vi "Initialize.vi"(8 "error in (no error)":errorcluster, 9 "Time":timestamp, 10 "Alias":string, 11 "NI DMM Calibration Data in":refnum<class "NI DMM Calibration Data.lvclass">) -> (0 "error out":errorcluster, 3 "NI DMM Calibration Data out":refnum<class "NI DMM Calibration Data.lvclass">)   [LabVIEW 2020, in "NI DMM Driver.lvlib" / "NI DMM Calibration Data.lvclass"]
doc: "Write Alias and Time and set all other values to NaN or FALSE."
uses:
  NI DMM Calibration Data.lvclass
  NI DMM Calibration Data.lvclass/NI DMM Calibration Data.ctl
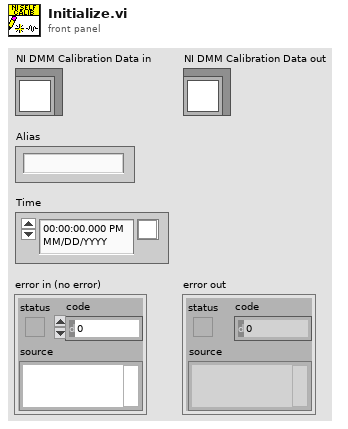
[diagram p1: front panel]
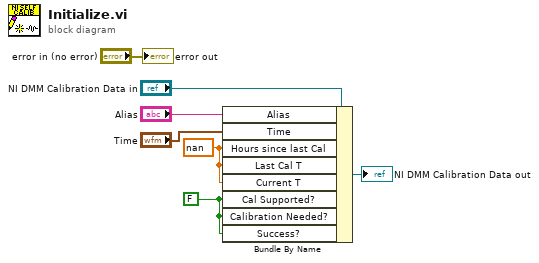
[diagram p0: block diagram]
diagram:
  w1 = FALSE ("Cal Supported?")
  w2 = nan ("Hours since last Cal")
  n1 = Bundle By Name(cluster="NI DMM Calibration Data in", "Alias"="Alias", "Time"="Time", "Hours since last Cal"=w2, "Last Cal T"=w2, "Current T"=w2, "Cal Supported?"=w1, "Calibration Needed?"=w1, "Success?"=w1) -> (→"NI DMM Calibration Data out":refnum<class "NI DMM Calibration Data.lvclass">)
  "error out" <- "error in (no error)"
